vi "Update Button Text.vi"(8 "Error In":errorcluster, 10 "Button Text":string="Working...", 11 "Button Ref":refnum<vi>) -> (0 "Error Out":errorcluster, 3 "Buffon Ref":refnum<vi>)   [LabVIEW 2014, in "LMH-LINX.lvlib"]
uses:
  <vilib>/MakerHub/LINX/LMH-LINX.lvlib
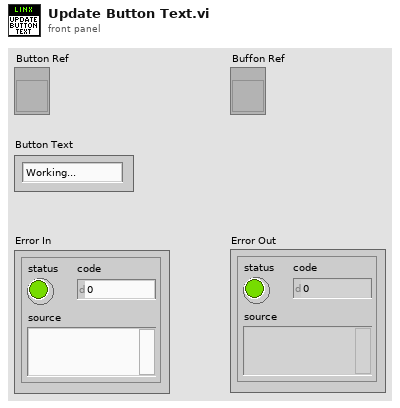
[diagram p1: front panel]
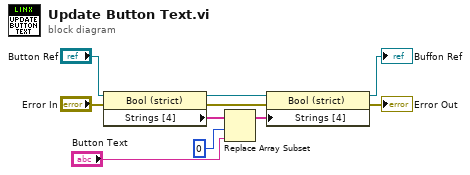
[diagram p0: block diagram]
diagram:
  n1 = property class="Bool (strict)"(reference="Button Ref", error in="Error In") -> (reference out=w5:refnum<vi>, error out=w6:errorcluster, "Strings [4]"=w2:string[])
  n2 = Replace Array Subset(array=w2, new element="Button Text", index=0) -> (w7:string[])
  n3 = property class="Bool (strict)"(reference=w5, error in=w6, "Strings [4]"=w7) -> (reference out=→"Buffon Ref":refnum<vi>, error out=→"Error Out":errorcluster)
